vi "loadAndFormatValues.vi"(5 "error in (no error)":errorcluster, 7 "configuration":T1, 9 "channel names":string[](array[string]), 10 "group names":string[](array[string]), 11 "tdms file":refnum<k34>) -> (0 "error out":errorcluster, 1 "graph y names":string, 2 "graph x names":string, 3 "tdms file out":refnum<k34>, 4 "waveform values":waveform(dbl)[](array[waveform]), 6 "table values":string[][](array[string]), 8 "table headers":string[](array[string]))   [LabVIEW 2017]
uses:
  <vilib>/Utility/tdmsutil.llb/fileViewerConfigData.ctl
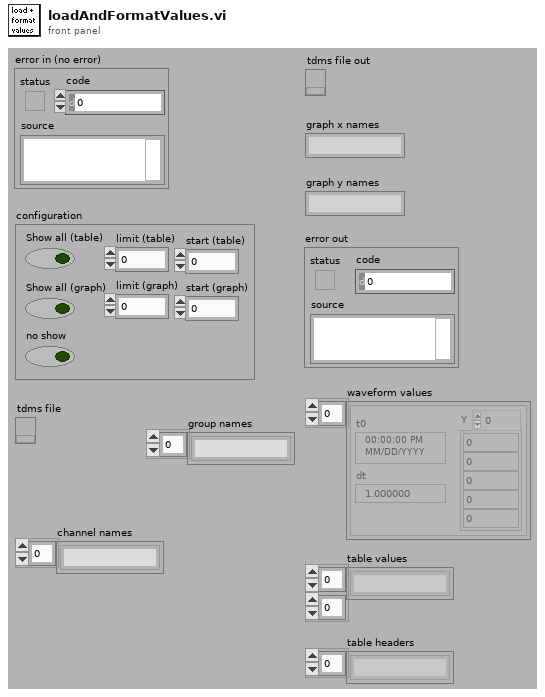
[diagram p1: front panel]
types:
  T1 = typedef "fileViewerConfigData.ctl" = cluster{"Show all (table)":bool, "Show all (graph)":bool, "limit (table)":u64, "limit (graph)":u64, "no show":bool, "start (table)":u64, "start (graph)":u64}
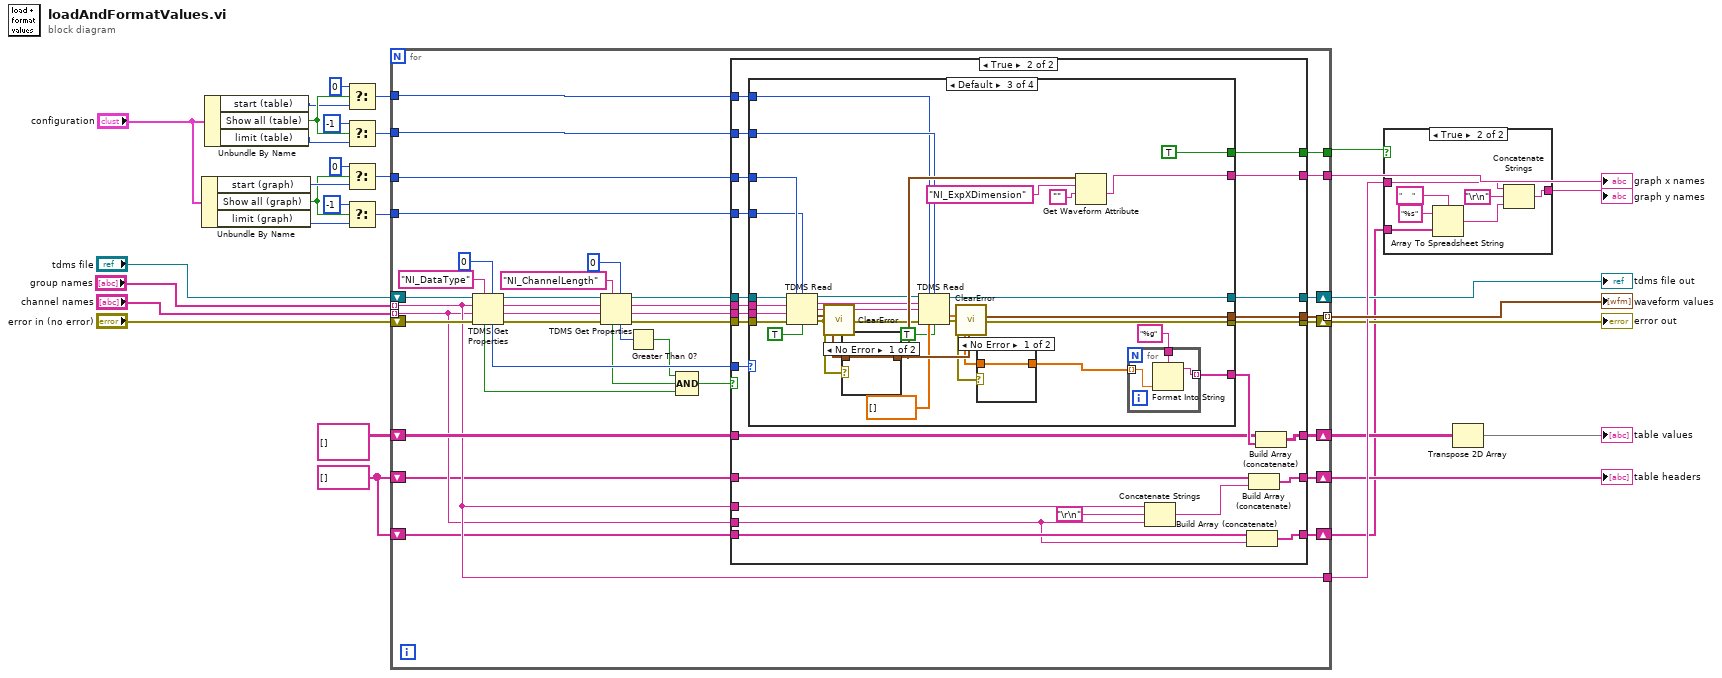
[diagram p0: block diagram]
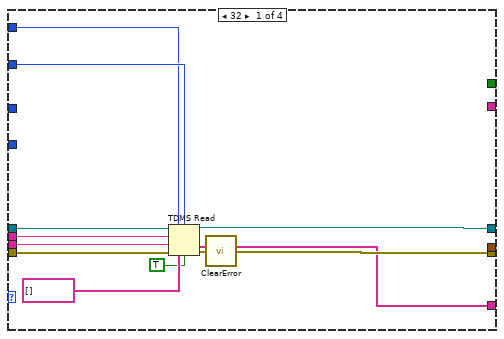
[diagram p4: hidden frame]
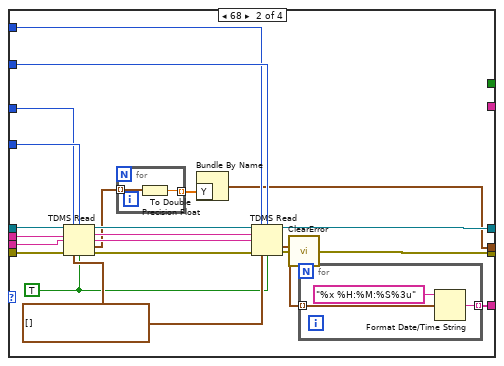
[diagram p5: hidden frame]
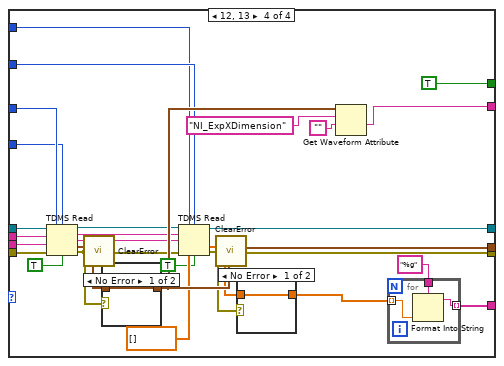
[diagram p8: hidden frame]
diagram:
  w1 = string[] []
  n1 = Unbundle By Name("configuration") -> ("start (graph)"=w27:u64, "Show all (graph)"=w26:bool, "limit (graph)"=w25:u64)
  n2 = Unbundle By Name("configuration") -> ("start (table)"=w20:u64, "Show all (table)"=w21:bool, "limit (table)"=w22:u64)
  n3 = Select(t=u64 0, s=w21, f=w20) -> (s? t:f=w23:u64)
  n4 = Select(t=i64 -1 ("count (-1: all)"), s=w21, f=w22) -> (s? t:f=w24:u64)
  n5 = Select(t=u64 0, s=w26, f=w27) -> (s? t:f=w31:u64)
  n6 = Select(t=i64 -1 ("count (-1: all)"), s=w26, f=w25) -> (s? t:f=w30:u64)
  n7 = for {
    tunnel: w31 -> [w68]
    tunnel: w30 -> [w67]
    tunnel: [w65] -> w14 mode=indexing
    tunnel: "channel names" -> [w37] mode=indexing
    shift-right: [w66] -> w9
    shift-left: "error in (no error)" -> [w63]
    shift-right: [w69] -> w7
    shift-left: "tdms file" -> [w62]
    tunnel: "group names" -> [w38] mode=indexing
    tunnel: [w64] -> w12
    tunnel: [w38] -> w10
    tunnel: [w58] -> w13
    tunnel: w24 -> [w57]
    tunnel: w23 -> [w56]
    shift-right: [w39] -> w5
    shift-left: string[][] [] -> [w40]
    shift-right: [w35] -> w3
    shift-left: w1 -> [w36]
    shift-right: [w33] -> w2
    shift-left: w1 -> [w34]
    n8 = TDMS Get Properties(5:u16 0, 7:"NI_DataType" ("property name"), 8:w63, 9:w37, 10:w38, 11:w62) -> (0:w55:errorcluster, 1:w48:string, 2:w49:string, 3:w54:refnum<k34>, 4:w59:u16, 6:w42:bool)
    n9 = TDMS Get Properties(5:u64 0, 7:"NI_ChannelLength" ("property name"), 8:w55, 9:w48, 10:w49, 11:w54) -> (0:w53:errorcluster, 1:w52:string, 2:w51:string, 3:w50:refnum<k34>, 4:w45:u64, 6:w43:bool)
    n10 = Greater Than 0?(x=w45) -> (x > 0?=w44:bool)
    n11 = Compound Arithmetic op=AND(w44, w43, w42) -> (w41:bool)
    n12 = case shown="True" w41 {
      tunnel: [w74 w99] -> w69
      tunnel: w68 -> [_ w98]
      tunnel: w67 -> [_ w97]
      tunnel: [w73 w87] -> w66
      tunnel: [_ w86] -> w65
      tunnel: [_ w96] -> w64
      tunnel: w50 -> [w74 w95]
      tunnel: w53 -> [w73 w94]
      tunnel: w51 -> [_ w93]
      tunnel: w52 -> [_ w92]
      tunnel: w59 -> [_ w91]
      tunnel: [_ w90] -> w58
      tunnel: w57 -> [_ w89]
      tunnel: w56 -> [_ w88]
      tunnel: w40 -> [w72 w83]
      tunnel: [w72 w84] -> w39
      tunnel: w38 -> [_ w81]
      tunnel: w37 -> [_ w76]
      tunnel: w36 -> [w71 w80]
      tunnel: [w71 w78] -> w35
      tunnel: w34 -> [w70 w77]
      tunnel: [w70 w75] -> w33
      frame False {
      }
      frame True {
        n13 = case shown="Default" w91 {
          tunnel: [w105 w132 w149 w183] -> w99
          tunnel: w98 -> [_ w116 w167 w201]
          tunnel: w97 -> [_ w117 w166 w200]
          tunnel: [w106 w133 w150 w184] -> w87
          tunnel: [w104 w131 w142 w176] -> w85
          tunnel: [_ w113 w157 w191] -> w86
          tunnel: [_ _ w139 w173] -> w96
          tunnel: w95 -> [w111 w125 w163 w197]
          tunnel: w94 -> [w108 w126 w162 w196]
          tunnel: w93 -> [w110 w124 w161 w195]
          tunnel: w92 -> [w109 w123 w160 w194]
          tunnel: [_ _ TRUE TRUE] -> w90
          tunnel: w89 -> [w103 w129 w148 w182]
          tunnel: w88 -> [w102 w128 w147 w181]
          frame 32 {
            n14 = TDMS Read(0:w111, 1:w102, 2:w103, 5:w110, 7:w109, 11:w108, 12:string[] [], 13:TRUE ("return channels in file order? (F)")) -> (4:w105:refnum<k34>, 10:w104:string[], 15:w101:errorcluster)  [unwired: 3 out]
            n15 = call <vilib>:"ClearError.vi"("error in (no error)"=w101) -> ("error out"=w106:errorcluster)
          }
          frame 68 {
            w118 = TRUE ("return channels in file order? (F)")
            w119 = timestamp[] []
            n16 = TDMS Read(0:w125, 1:w116, 2:w117, 5:w124, 7:w123, 11:w126, 12:w119, 13:w118) -> (4:w120:refnum<k34>, 6:w121:string, 8:w122:string, 10:w115:timestamp[], 15:w112:errorcluster)  [unwired: 1 out]
            n17 = for {
              tunnel: w115 -> [w135] mode=indexing
              tunnel: [w134] -> w114 mode=indexing
              n18 = To Double Precision Float(number=w135) -> (double precision float=w134:dbl)
            }
            n19 = Bundle By Name("Y"=w114) -> (w113:waveform(dbl))  [unwired: 1 in]
            n20 = TDMS Read(0:w120, 1:w128, 2:w129, 5:w121, 7:w122, 11:w112, 12:w119, 13:w118) -> (4:w132:refnum<k34>, 10:w130:timestamp[], 15:w127:errorcluster)  [unwired: 3 out]
            n21 = call <vilib>:"ClearError.vi"("error in (no error)"=w127) -> ("error out"=w133:errorcluster)
            n22 = for {
              tunnel: [w138] -> w131 mode=indexing
              tunnel: w130 -> [w137] mode=indexing
              n23 = Format Date/Time String(time format string (%c)="%x %H:%M:%S%3u", seconds (now)=w137) -> (date/time string=w138:string)  [unwired: 1 in]
            }
          }
          frame Default {
            n24 = TDMS Read(0:w163, 1:w167, 2:w166, 5:w161, 7:w160, 11:w162, 13:TRUE ("return channels in file order? (F)")) -> (4:w156:refnum<k34>, 6:w154:string, 8:w153:string, 10:w158:waveform(dbl), 15:w145:errorcluster)  [unwired: 1 in, 1 out]
            n25 = call <vilib>:"ClearError.vi"("error in (no error)"=w145) -> ("error out"=w155:errorcluster)
            n26 = case shown="No Error" w155 {
              tunnel: w158 -> [w172 _]
              tunnel: [w172 _] -> w157
              frame No Error {
              }
              frame Error {
              }
            }
            n27 = TDMS Read(0:w156, 1:w147, 2:w148, 5:w154, 7:w153, 11:w155, 12:dbl[] [], 13:TRUE ("return channels in file order? (F)")) -> (4:w149:refnum<k34>, 10:w152:dbl[], 15:w146:errorcluster)  [unwired: 3 out]
            n28 = call <vilib>:"ClearError.vi"("error in (no error)"=w146) -> ("error out"=w150:errorcluster)
            n29 = case shown="No Error" w150 {
              tunnel: w152 -> [w171 _]
              tunnel: [w171 _] -> w143
              frame No Error {
              }
              frame Error {
              }
            }
            n30 = Get Waveform Attribute(5:"", 6:"NI_ExpXDimension" ("name"), 7:w157) -> (1:w139:string)  [unwired: 1 in, 3 out]
            n31 = for {
              tunnel: "%g" ("format string") -> [w170]
              tunnel: w143 -> [w169] mode=indexing
              tunnel: [w168] -> w142 mode=indexing
              n32 = Format Into String(format string=w170, w169) -> (resulting string=w168:string)  [unwired: 2 in, 1 out]
            }
          }
          frame 12, 13 {
            n33 = TDMS Read(0:w197, 1:w201, 2:w200, 5:w195, 7:w194, 11:w196, 13:TRUE ("return channels in file order? (F)")) -> (4:w190:refnum<k34>, 6:w188:string, 8:w187:string, 10:w192:waveform(dbl), 15:w179:errorcluster)  [unwired: 1 in, 1 out]
            n34 = call <vilib>:"ClearError.vi"("error in (no error)"=w179) -> ("error out"=w189:errorcluster)
            n35 = case shown="No Error" w189 {
              tunnel: w192 -> [w206 _]
              tunnel: [w206 _] -> w191
              frame No Error {
              }
              frame Error {
              }
            }
            n36 = TDMS Read(0:w190, 1:w181, 2:w182, 5:w188, 7:w187, 11:w189, 12:cdb[] [], 13:TRUE ("return channels in file order? (F)")) -> (4:w183:refnum<k34>, 10:w186:cdb[], 15:w180:errorcluster)  [unwired: 3 out]
            n37 = call <vilib>:"ClearError.vi"("error in (no error)"=w180) -> ("error out"=w184:errorcluster)
            n38 = case shown="No Error" w184 {
              tunnel: w186 -> [w205 _]
              tunnel: [w205 _] -> w177
              frame No Error {
              }
              frame Error {
              }
            }
            n39 = Get Waveform Attribute(5:"", 6:"NI_ExpXDimension" ("name"), 7:w191) -> (1:w173:string)  [unwired: 1 in, 3 out]
            n40 = for {
              tunnel: "%g" ("format string") -> [w204]
              tunnel: w177 -> [w203] mode=indexing
              tunnel: [w202] -> w176 mode=indexing
              n41 = Format Into String(format string=w204, w203) -> (resulting string=w202:string)  [unwired: 2 in, 1 out]
            }
          }
        }
        n42 = Concatenate Strings(w81, "\r\n", w76) -> (w79:string)
        n43 = Build Array (concatenate)(w77, w76) -> (w75:string[])
        n44 = Build Array (concatenate)(w80, w79) -> (w78:string[])
        n45 = Build Array (concatenate)(w83, w85) -> (w84:string[][])
      }
    }
  }
  "waveform values" <- w14
  "graph x names" <- w12
  "table headers" <- w3
  "error out" <- w9
  "tdms file out" <- w7
  n46 = case shown="True" w13 {
    tunnel: w2 -> [_ w212]
    tunnel: w10 -> [_ w209]
    tunnel: [_ w208] -> w11
    frame False {
    }
    frame True {
      n47 = Array To Spreadsheet String(delimiter (Tab)="     ", array=w212, 3:"%s" ("format string")) -> (spreadsheet string=w210:string)
      n48 = Concatenate Strings(w209, "\r\n", w210) -> (w208:string)
    }
  }
  "graph y names" <- w11
  n49 = Transpose 2D Array(2D array=w5) -> (transposed array=→"table values":string[][])
